vi "get properties.vi"(8 "error in (no error)":errorcluster, 11 "Camera":T2) -> (0 "error out":errorcluster, 2 "Properties":T1(array[cluster]), 3 "Camera out":T2)   [LabVIEW 2022 SP3, in "Vision.lvlib"]
uses:
  Vision.lvlib
  camera.ctl
  camera driver.ctl
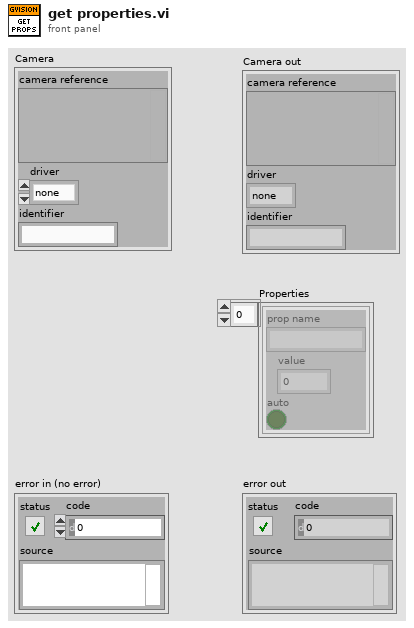
[diagram p1: front panel]
types:
  T1 = cluster{"prop name":string, "value":sgl, "auto":bool}[]
  T2 = typedef "Vision.lvlib/camera.ctl" = cluster{"camera reference":variant, "driver":T3, "identifier":string}
  T3 = typedef "Vision.lvlib/camera driver.ctl" = enum16{"none", "ueye", "wmf", "imaqdx"}
  T4 = cluster{"prop name":string, "value":sgl, "auto":bool}
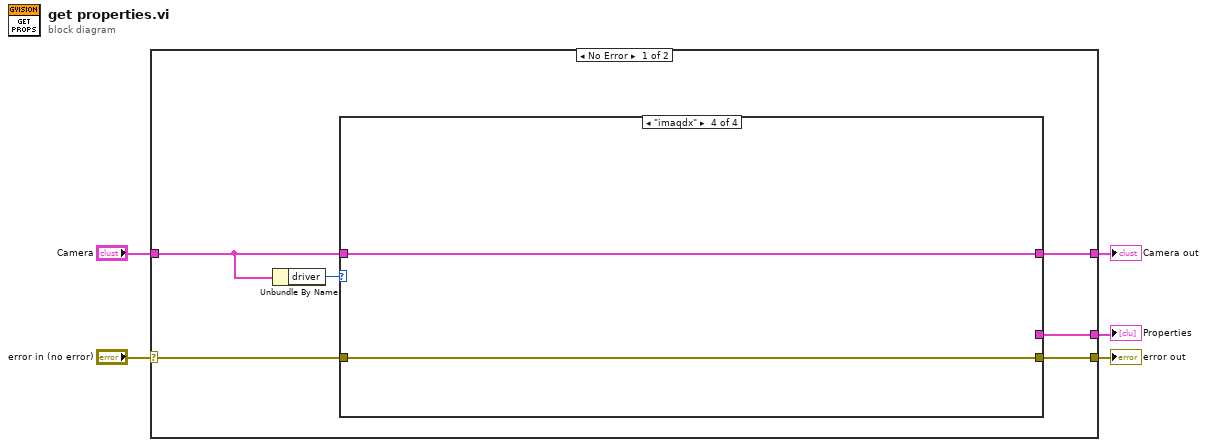
[diagram p0: block diagram]
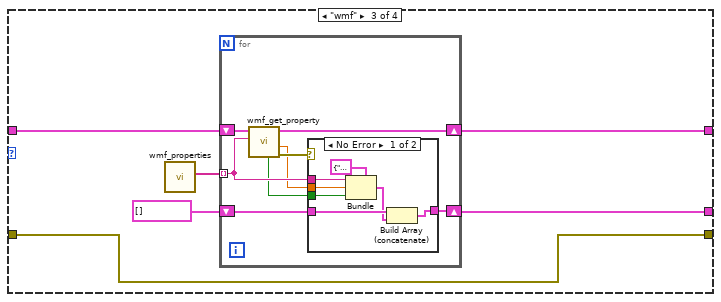
[diagram p4: hidden frame]
diagram:
  n1 = case shown="No Error" "error in (no error)" {
    selector: "error in (no error)" -> [w9 w41]
    tunnel: [w10 w41] -> w4
    tunnel: "Camera" -> [w8 w40]
    tunnel: [w7 w40] -> w2
    tunnel: [w6 _] -> w1
    frame No Error {
      n2 = Unbundle By Name(w8) -> ("driver"=w11:T3)
      n3 = case shown="\"imaqdx\"" w11 {
        tunnel: w9 -> [w13 w15 w16 w39]
        tunnel: [w13 w15 w16 w39] -> w10
        tunnel: w8 -> [w12 w14 w20 w38]
        tunnel: [w12 w14 w18 w38] -> w7
        tunnel: [_ _ w17 _] -> w6
        frame "none" {
        }
        frame "ueye" {
        }
        frame "wmf" {
          n4 = call "wmf_properties.vi"() -> ("WMF Properties"=w21:string[])  [unwired: 11 in]
          n5 = for {
            tunnel: w21 -> [w26] mode=indexing
            shift-right: [w22] -> w17
            shift-left: T1 [] -> [w27]
            shift-right: [w23] -> w18
            shift-left: w20 -> [w29]
            n6 = call "wmf_get_property.vi"("property name"=w26, "Camera"=w29) -> ("error out"=w28:errorcluster, "Value"=w24:sgl, "Camera out"=w23:T2, "Auto"=w25:bool)  [unwired: 6 in]
            n7 = case shown="No Error" w28 {
              tunnel: w27 -> [w36 w37]
              tunnel: w26 -> [w33 _]
              tunnel: w25 -> [w31 _]
              tunnel: w24 -> [w32 _]
              tunnel: [w30 w37] -> w22
              frame No Error {
                n8 = Bundle(cluster=T4 {"prop name"="", "value"=0.0, "auto"=TRUE}, "prop name"=w33, "value"=w32, "auto"=w31) -> (w34:T4)
                n9 = Build Array (concatenate)(w36, w34) -> (w30:T1)
              }
              frame Error {
              }
            }
          }
        }
        frame "imaqdx" {
        }
      }
    }
    frame Error {
    }
  }
  "error out" <- w4
  "Camera out" <- w2
  "Properties" <- w1
